vi "Client Synchronize Data.vi"(7 "force configure? (F)":bool, 8 "error in":errorcluster, 11 "connection ID in":T1) -> (0 "error out":errorcluster, 3 "connection ID out":T1)   [LabVIEW 2010, in "NI_CCC.lvlib"]
doc: "Sends the values of the write tag list to the CCC server, and requests the latest values of the read tag list from the server. This VI is equivalent to calling Client Write.vi and Client Read.vi consecutively, but it reduces the number of messages sent betwen the client and server."
uses:
  NI_CCC.lvlib
  Connection ID.ctl
  <vilib>/NI/STM/TCP/TCP Connection Info.ctl
  <vilib>/NI/STM/SubVIs/MetaDataElement.ctl
  Tag Configuration.ctl
  <vilib>/NI/Current Value Table/Type Defs/Data Types.ctl
  Tag Direction.ctl
  <vilib>/NI/STM/TCP/TCP Read Options.ctl
  <vilib>/NI/STM/TCP/TCP Write Options.ctl
  <vilib>/NI/Current Value Table/Type Defs/Group Data.ctl
  <vilib>/NI/Current Value Table/Write grouped data to tags.vi
  Read Error.vi
  Initialize Address_Index Lists.vi
  <vilib>/NI/Current Value Table/Read tags into grouped data.vi
  <vilib>/NI/Current Value Table/Write Index Set.vi
  <vilib>/NI/Current Value Table/DataTypes/Double_Write Index Set.vi
  <vilib>/NI/Current Value Table/DataTypes/Array of String_Write Index Set.vi
  <vilib>/NI/Current Value Table/DataTypes/Array of Boolean_Write Index Set.vi
  <vilib>/NI/Current Value Table/DataTypes/Array of Single_Write Index Set.vi
  <vilib>/NI/Current Value Table/DataTypes/Array of Double_Write Index Set.vi
  <vilib>/NI/Current Value Table/DataTypes/Array of I8_Write Index Set.vi
  <vilib>/NI/Current Value Table/DataTypes/Array of I16_Write Index Set.vi
  <vilib>/NI/Current Value Table/DataTypes/Array of I32_Write Index Set.vi
  <vilib>/NI/Current Value Table/DataTypes/Array of I64_Write Index Set.vi
  <vilib>/NI/Current Value Table/DataTypes/Array of U64_Write Index Set.vi
  <vilib>/NI/Current Value Table/DataTypes/Array of U32_Write Index Set.vi
  <vilib>/NI/Current Value Table/DataTypes/Array of U16_Write Index Set.vi
  <vilib>/NI/Current Value Table/DataTypes/Array of U8_Write Index Set.vi
  <vilib>/NI/Current Value Table/DataTypes/Boolean_Write Index Set.vi
  <vilib>/NI/Current Value Table/DataTypes/String_Write Index Set.vi
  <vilib>/NI/Current Value Table/DataTypes/U8_Write Index Set.vi
  <vilib>/NI/Current Value Table/DataTypes/U16_Write Index Set.vi
  <vilib>/NI/Current Value Table/DataTypes/U32_Write Index Set.vi
  <vilib>/NI/Current Value Table/DataTypes/U64_Write Index Set.vi
  <vilib>/NI/Current Value Table/DataTypes/I8_Write Index Set.vi
  <vilib>/NI/Current Value Table/DataTypes/I16_Write Index Set.vi
  <vilib>/NI/Current Value Table/DataTypes/I32_Write Index Set.vi
  <vilib>/NI/Current Value Table/DataTypes/I64_Write Index Set.vi
  <vilib>/NI/Current Value Table/DataTypes/Single_Write Index Set.vi
  <vilib>/NI/Current Value Table/Get Index and Type.vi
  <vilib>/NI/Current Value Table/Group Tags.vi
  <vilib>/NI/Current Value Table/Read Index Set.vi
  <vilib>/NI/Current Value Table/DataTypes/Double_Read Index Set.vi
  <vilib>/NI/Current Value Table/DataTypes/Array of String_Read Index Set.vi
  <vilib>/NI/Current Value Table/DataTypes/Array of Boolean_Read Index Set.vi
  <vilib>/NI/Current Value Table/DataTypes/Array of Single_Read Index Set.vi
  <vilib>/NI/Current Value Table/DataTypes/Array of Double_Read Index Set.vi
  <vilib>/NI/Current Value Table/DataTypes/Array of I8_Read Index Set.vi
  <vilib>/NI/Current Value Table/DataTypes/Array of I16_Read Index Set.vi
  <vilib>/NI/Current Value Table/DataTypes/Array of I32_Read Index Set.vi
  <vilib>/NI/Current Value Table/DataTypes/Array of I64_Read Index Set.vi
  <vilib>/NI/Current Value Table/DataTypes/Array of U64_Read Index Set.vi
  <vilib>/NI/Current Value Table/DataTypes/Array of U32_Read Index Set.vi
  <vilib>/NI/Current Value Table/DataTypes/Array of U16_Read Index Set.vi
  <vilib>/NI/Current Value Table/DataTypes/Array of U8_Read Index Set.vi
  <vilib>/NI/Current Value Table/DataTypes/Boolean_Read Index Set.vi
  <vilib>/NI/Current Value Table/DataTypes/String_Read Index Set.vi
  <vilib>/NI/Current Value Table/DataTypes/U8_Read Index Set.vi
  <vilib>/NI/Current Value Table/DataTypes/U16_Read Index Set.vi
  <vilib>/NI/Current Value Table/DataTypes/U32_Read Index Set.vi
  <vilib>/NI/Current Value Table/DataTypes/U64_Read Index Set.vi
  <vilib>/NI/Current Value Table/DataTypes/I8_Read Index Set.vi
  <vilib>/NI/Current Value Table/DataTypes/I16_Read Index Set.vi
  <vilib>/NI/Current Value Table/DataTypes/I32_Read Index Set.vi
  <vilib>/NI/Current Value Table/DataTypes/I64_Read Index Set.vi
  <vilib>/NI/Current Value Table/DataTypes/Single_Read Index Set.vi
  <vilib>/Utility/error.llb/Error Cluster From Error Code.vi
  FG Client Configurations.vi
  <vilib>/NI/Current Value Table/FGVs/Tag Memory.vi
  <vilib>/NI/Current Value Table/FGVs/Group Memory.vi
  <vilib>/NI/Current Value Table/Form Single Group.vi
  <vilib>/NI/Current Value Table/Memory Block.vi
  <vilib>/NI/Current Value Table/DataTypes/Double_Memory Block.vi
  <vilib>/NI/Current Value Table/DataTypes/Array of String_Memory Block.vi
  <vilib>/NI/Current Value Table/DataTypes/Array of Boolean_Memory Block.vi
  <vilib>/NI/Current Value Table/DataTypes/Array of Single_Memory Block.vi
  <vilib>/NI/Current Value Table/DataTypes/Array of Double_Memory Block.vi
  <vilib>/NI/Current Value Table/DataTypes/Array of I8_Memory Block.vi
  <vilib>/NI/Current Value Table/DataTypes/Array of I16_Memory Block.vi
  <vilib>/NI/Current Value Table/DataTypes/Array of I32_Memory Block.vi
  <vilib>/NI/Current Value Table/DataTypes/Array of I64_Memory Block.vi
  <vilib>/NI/Current Value Table/DataTypes/Array of U64_Memory Block.vi
  <vilib>/NI/Current Value Table/DataTypes/Array of U32_Memory Block.vi
  <vilib>/NI/Current Value Table/DataTypes/Array of U16_Memory Block.vi
  <vilib>/NI/Current Value Table/DataTypes/Array of U8_Memory Block.vi
  <vilib>/NI/Current Value Table/DataTypes/Boolean_Memory Block.vi
  <vilib>/NI/Current Value Table/DataTypes/String_Memory Block.vi
  <vilib>/NI/Current Value Table/DataTypes/U8_Memory Block.vi
  <vilib>/NI/Current Value Table/DataTypes/U16_Memory Block.vi
  <vilib>/NI/Current Value Table/DataTypes/U32_Memory Block.vi
  <vilib>/NI/Current Value Table/DataTypes/U64_Memory Block.vi
  <vilib>/NI/Current Value Table/DataTypes/I8_Memory Block.vi
  <vilib>/NI/Current Value Table/DataTypes/I16_Memory Block.vi
  <vilib>/NI/Current Value Table/DataTypes/I32_Memory Block.vi
  <vilib>/NI/Current Value Table/DataTypes/I64_Memory Block.vi
  <vilib>/NI/Current Value Table/DataTypes/Single_Memory Block.vi
  <vilib>/NI/STM/NI STM.lvlib
  <vilib>/NI/Current Value Table/Current Value Table.lvlib
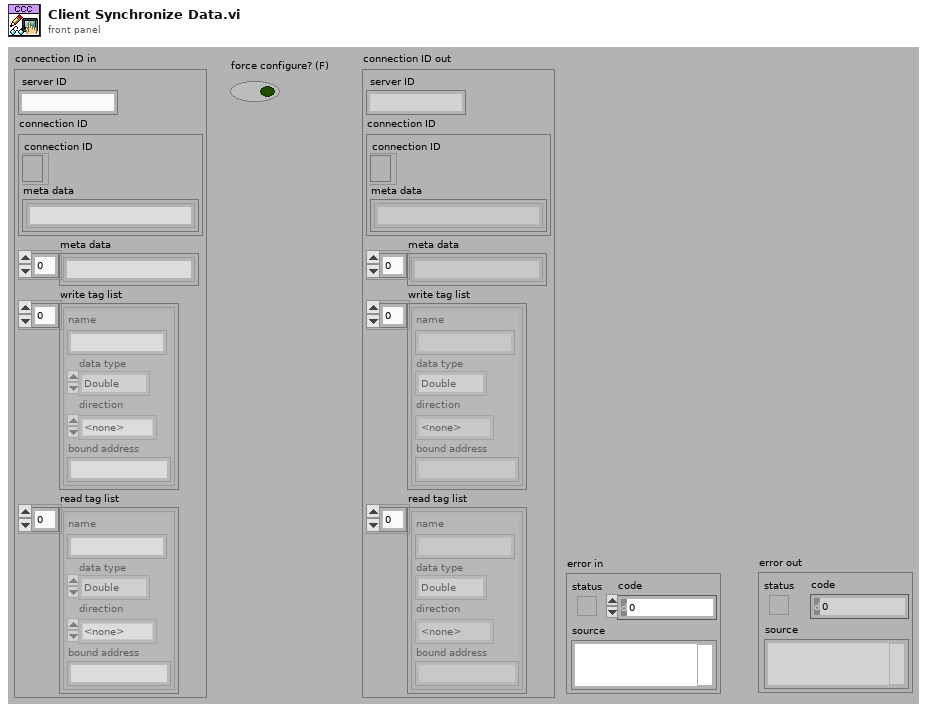
[diagram p1: front panel]
types:
  T1 = typedef "NI_CCC.lvlib/Connection ID.ctl" = cluster{"server ID":string, "connection ID":T2, "meta data":T3[], "write tag list":T4[], "read tag list":T4[]}
  T2 = typedef "NI STM.lvlib/TCP Connection Info.ctl" = cluster{"connection ID":refnum<k5>, "meta data":T3[]}
  T3 = typedef "NI STM.lvlib/MetaDataElement.ctl" = string
  T4 = typedef "NI_CCC.lvlib/Tag Configuration.ctl" = cluster{"name":string, "data type":T5, "direction":T6, "bound address":string}
  T5 = typedef "Current Value Table.lvlib/Data Types.ctl" = enum16{"Double", "Single", "I64", "I32", "I16", "I8", "U64", "U32", "U16", "U8", "String", "Boolean", "Array of U8", "Array of U16", "Array of U32", "Array of U64", "Array of I64", "Array of I32", "Array of I16", "Array of I8", "Array of Double", "Array of Single", "Array of Boolean", "Array of String"}
  T6 = typedef "NI_CCC.lvlib/Tag Direction.ctl" = enum32{"<none>", "Read", "Write"}
  T7 = typedef "NI STM.lvlib/TCP Read Options.ctl" = cluster{"ignore timeout error":bool, "timeout ms (1000)":i32}
  T8 = typedef "NI STM.lvlib/TCP Write Options.ctl" = cluster{"ignore timeout error":bool, "timeout ms (1000)":i32}
  T9 = typedef "Current Value Table.lvlib/Group Data.ctl" = cluster{"Double":dbl[], "Single":sgl[], "I64":i64[], "I32":i32[], "I16":i16[], "I8":i8[], "U64":u64[], "U32":u32[], "U16":u16[], "U8":u8[], "String":string[], "Boolean":bool[], "Array of U8":cluster{"U8 Array":u8[]}[], "Array of U16":cluster{"U16 Array":u16[]}[], "Array of U32":cluster{"U32 Array":u32[]}[], "Array of U64":cluster{"U64 Array":u64[]}[], "Array of I64":cluster{"I64 Array":i64[]}[], "Array of I32":cluster{"I32 Array":i32[]}[], "Array of I16":cluster{"I16 Array":i16[]}[], "Array of I8":cluster{"I8 Array":i8[]}[], "Array of Double":cluster{"DBL Array":dbl[]}[], "Array of Single":cluster{"SGL Array":sgl[]}[], "Array of Boolean":cluster{"Boolean Array":bool[]}[], "Array of String":cluster{"String Array":string[]}[]}
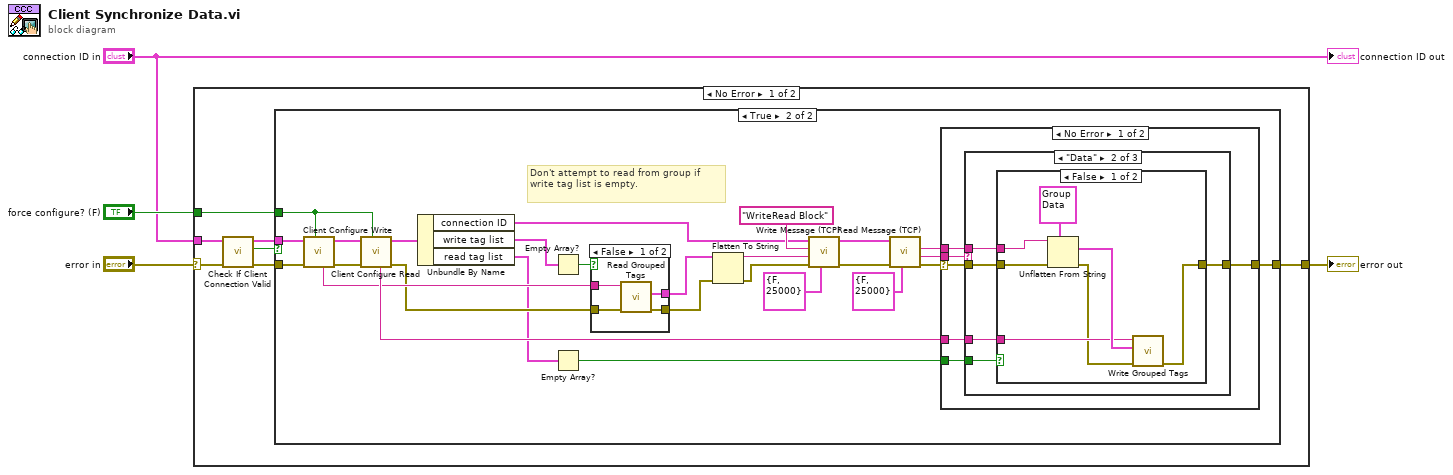
[diagram p0: block diagram]
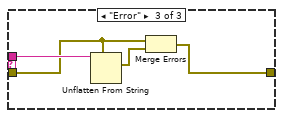
[diagram p6: hidden frame]
diagram:
  n1 = case shown="No Error" "error in" {
    selector: "error in" -> [w6 w70]
    tunnel: [w11 w70] -> w4
    tunnel: "force configure? (F)" -> [w10 _]
    tunnel: "connection ID in" -> [w9 _]
    frame No Error {
      n2 = call "Check If Client Connection Valid.vi"("error in"=w6, "connection ID in"=w9) -> ("error out"=w5:errorcluster, "valid?"=w8:bool, "connection ID out"=w7:T1)  [unwired: 7 in]
      n3 = case shown="True" w8 {
        tunnel: [w12 w33] -> w11
        tunnel: w5 -> [w12 w25]
        tunnel: w10 -> [_ w23]
        tunnel: w7 -> [_ w27]
        frame False {
        }
        frame True {
          # "Don't attempt to read from group if write tag list is empty."
          n4 = call "Client Configure Write.vi"("force configure? (F)"=w23, "error in"=w25, "connection ID in"=w27) -> ("error out"=w24:errorcluster, "connection ID out"=w26:T1, "write group name"=w22:string)  [unwired: 5 in, 1 out]
          n5 = call "Client Configure Read.vi"("force configure? (F)"=w23, "error in"=w24, "connection ID in"=w26) -> ("error out"=w21:errorcluster, "connection ID out"=w28:T1, "read group name"=w30:string)  [unwired: 5 in, 1 out]
          n6 = Unbundle By Name(w28) -> ("connection ID"=w29:T2, "write tag list"=w16:T4[], "read tag list"=w14:T4[])
          n7 = Empty Array?(array=w16) -> (empty?=w15:bool)
          n8 = Empty Array?(array=w14) -> (empty?=w13:bool)
          n9 = case shown="False" w15 {
            tunnel: w22 -> [w43 _]
            tunnel: w21 -> [w42 w44]
            tunnel: [w41 _] -> w20
            tunnel: [w40 w44] -> w19
            frame False {
              n10 = call <vilib>:"Read Grouped Tags.vi"("error in (no error)"=w42, "Group"=w43) -> ("error out"=w40:errorcluster, "Data"=w41:T9)  [unwired: 8 in]
            }
            frame True {
            }
          }
          n11 = Flatten To String(anything=w20, error in (no error)=w19) -> (data string=w18:string, error out=w17:errorcluster)  [unwired: 3 out]
          n12 = call <vilib>:"Write Message (TCP).vi"("options"=T8 {"ignore timeout error"=FALSE, "timeout ms (1000)"=25000} ("Options"), "error in"=w17, "data"=w18, "name"="WriteRead Block" ("Name"), "connection info in"=w29) -> ("error out"=w36:errorcluster, "connection info out"=w35:T2)  [unwired: 5 in]
          n13 = call <vilib>:"Read Message (TCP).vi"("options"=T7 {"ignore timeout error"=FALSE, "timeout ms (1000)"=25000} ("Options"), "error in"=w36, "connection info in"=w35) -> ("error out"=w34:errorcluster, "name"=w38:T3, "data string"=w37:string)  [unwired: 3 in, 3 out]
          n14 = case shown="No Error" w34 {
            selector: w34 -> [w50 w69]
            tunnel: w38 -> [w49 _]
            tunnel: w37 -> [w48 _]
            tunnel: [w46 w69] -> w33
            tunnel: w30 -> [w47 _]
            tunnel: w13 -> [w45 _]
            frame No Error {
              n15 = case shown="\"Data\"" w49 {
                tunnel: w48 -> [_ w56 w68]
                tunnel: w50 -> [w51 w55 w67]
                tunnel: [w51 w53 w66] -> w46
                tunnel: w47 -> [_ w54 _]
                tunnel: w45 -> [_ w52 _]
                frame Default {
                  # "Unexpected Command"
                }
                frame "Data" {
                  n16 = case shown="False" w52 {
                    tunnel: w56 -> [w63 _]
                    tunnel: w55 -> [w62 w64]
                    tunnel: w54 -> [w59 _]
                    tunnel: [w57 w64] -> w53
                    frame False {
                      n17 = Unflatten From String(type=T9 {"Double"=[], "Single"=[], "I64"=[], "I32"=[], "I16"=[], "I8"=[], "U64"=[], "U32"=[], "U16"=[], "U8"=[], "String"=[], "Boolean"=[], "Array of U8"=[], "Array of U16"=[], "Array of U32"=[], "Array of U64"=[], "Array of I64"=[], "Array of I32"=[], "Array of I16"=[], "Array of I8"=[], "Array of Double"=[], "Array of Single"=[], "Array of Boolean"=[], "Array of String"=[]} ("Data"), binary string=w63, error in (no error)=w62) -> (value=w60:T9, error out=w58:errorcluster)  [unwired: 3 out]
                      n18 = call <vilib>:"Write Grouped Tags.vi"("error in (no error)"=w58, "Data"=w60, "Group"=w59) -> ("error out"=w57:errorcluster)  [unwired: 8 in]
                    }
                    frame True {
                      # "Don't attempt to write to group if read tag list is empty."
                    }
                  }
                }
                frame "Error" {
                  n19 = Unflatten From String(type=w67, binary string=w68) -> (value=w65:errorcluster)  [unwired: 1 in, 4 out]
                  n20 = Merge Errors(w67, w65) -> (w66:errorcluster)
                }
              }
            }
            frame Error {
            }
          }
        }
      }
    }
    frame Error {
    }
  }
  "error out" <- w4
  "connection ID out" <- "connection ID in"
